vi "P4CMD Dialog_HistActDesc.vi"(8 "revision index (0)":i32, 9 "depot file index (0)":i32, 11 "history array":cluster{string[][], string[]}[](array[cluster])) -> (0 "file type":string, 2 "action":string, 3 "revision data":string[][](array[string]), 4 "description":string)   [LabVIEW 2020, in "NI_SCC_P4CMD.lvlib"]
uses:
  <vilib>/SourceControl/Providers/P4CMD/NI_SCC_P4CMD.lvlib
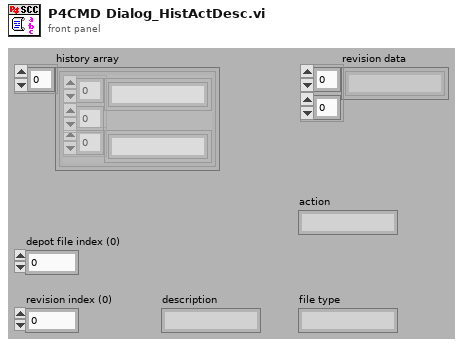
[diagram p1: front panel]
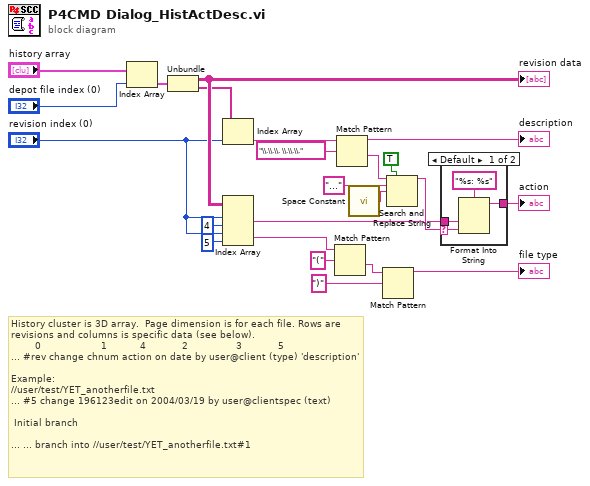
[diagram p0: block diagram]
diagram:
  # "History cluster is 3D array.  Page dimension is for each file. Rows are revisions and columns is specific data (see below).\n        0                    1           4            2                3            5\n... #rev change chnum action on date by user@client (type) 'description'\n\nExample:\n//user/test/YET_anotherfile.txt\n... #5 change 196123edit on 2004/03/19 by user@clientspec (text)\n\n\tInitial branch\n\n... ... branch into //user/test/YET_anotherfile.txt#1"
  n1 = Index Array(array="history array", index="depot file index (0)") -> (element=w5:cluster{string[][], string[]})
  n2 = Unbundle(w5) -> (w19:string[][], w6:string[])
  "revision data" <- w19
  n3 = Index Array(array=w6, index="revision index (0)") -> (element=w10:string)
  n4 = Index Array(array=w19, index (row) #1="revision index (0)", index (col) #1=4 ("disabled index (col)"), index (row) #2="revision index (0)", index (col) #2=5 ("disabled index (col)")) -> (element #1=w8:string, element #2=w1:string)
  n5 = Match Pattern(string=w1, regular expression="(") -> (after substring=w23:string)  [unwired: 1 in, 3 out]
  n6 = Match Pattern(string=w10, regular expression="\\.\\.\\. \\.\\.\\.") -> (before substring=→"description":string, after substring=w12:string)  [unwired: 1 in, 2 out]
  n7 = call <vilib>:"Space Constant.vi"() -> ("String"=w14:string)
  n8 = Match Pattern(string=w23, regular expression=")") -> (before substring=→"file type":string)  [unwired: 1 in, 3 out]
  n9 = Search and Replace String(replace all?=TRUE ("replace all? (F)"), input string=w12, search string="..." ("regular expression"), replace string=w14) -> (result string=w17:string)  [unwired: 4 in, 3 out]
  n10 = case shown="Default" w17 {
    selector: w17 -> [w24 _]
    tunnel: w8 -> [w26 w28]
    tunnel: [w25 w28] -> w16
    frame Default {
      n11 = Format Into String(format string="%s: %s", w26, w24) -> (resulting string=w25:string)  [unwired: 2 in, 1 out]
    }
    frame "" {
    }
  }
  "action" <- w16
